vi "util_multiline_int_to_array.vi"(1 "Multiline integer string":string) -> (0 "Array":i32[](array[numeric]))   [LabVIEW 2016]
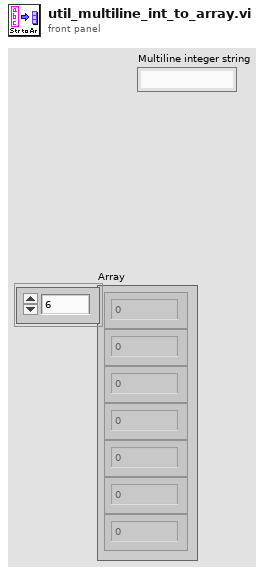
[diagram p1: front panel]
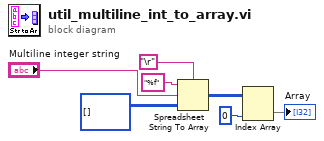
[diagram p0: block diagram]
diagram:
  n1 = Spreadsheet String To Array(delimiter (Tab)="\r", format string="%f", spreadsheet string="Multiline integer string", array type (2D Dbl)=i32[][] []) -> (array=w5:i32[][])
  n2 = Index Array(array=w5, index (col)=0 ("index (row)")) -> (element=→"Array":i32[])  [unwired: 1 in]
